vi "LibXML_GetNodeXMLText.vi"(8 "error in":errorcluster, 10 "xmlNodePtr":u32, 11 "xmlDocPtr":u32) -> (0 "error out":errorcluster, 3 "XMLString":string)   [LabVIEW 2019, in "Tools.lvlib"]
doc: "Gets the raw XML text of any node."
uses:
  Tools.lvlib
  dll/libxml2.dll
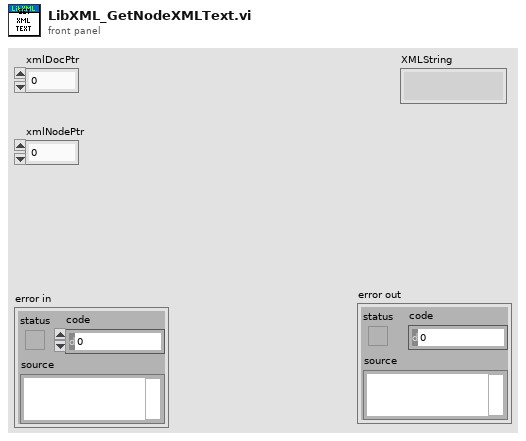
[diagram p1: front panel]
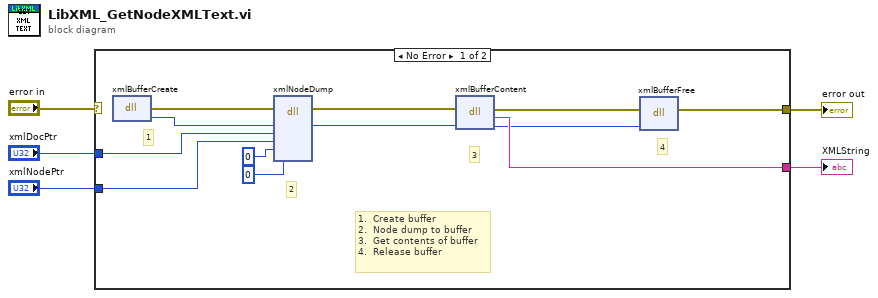
[diagram p0: block diagram]
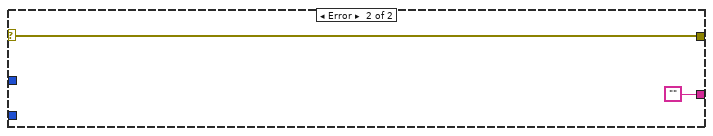
[diagram p2: hidden frame]
diagram:
  n1 = case shown="No Error" "error in" {
    selector: "error in" -> [_ w19]
    tunnel: "xmlDocPtr" -> [w15 _]
    tunnel: "xmlNodePtr" -> [w14 _]
    tunnel: [w11 ""] -> w3
    tunnel: [w6 w19] -> w2
    frame No Error {
      # "4"
      # "3"
      # "2"
      # "1"
      # "1.  Create buffer\n2.  Node dump to buffer\n3.  Get contents of buffer\n4.  Release buffer"
      n2 = dll-call lib="C:/Projects/_Prywatne/MyCIT/Framework/Tools/XML/LibXML/dll/libxml2.dll" fn="xmlBufferCreate"() -> (error out=w16:errorcluster, "xmlBufferPtr"=w17:u32)  [unwired: 3 in, 1 out]
      n3 = dll-call lib="C:/Projects/_Prywatne/MyCIT/Framework/Tools/XML/LibXML/dll/libxml2.dll" fn="xmlNodeDump"(error in=w16, "xmlBufferPtr"=w17, "xmlDocPtr"=w15, "xmlNodePtr"=w14, "level"=0, "format"=0) -> (error out=w12:errorcluster, "xmlBufferPtr"=w13:u32)  [unwired: 7 in, 1 out]
      n4 = dll-call lib="C:/Projects/_Prywatne/MyCIT/Framework/Tools/XML/LibXML/dll/libxml2.dll" fn="xmlBufferContent"(error in=w12, "xmlBufferPtr"=w13) -> (error out=w9:errorcluster, "XMLString"=w11:string, "xmlBufferPtr"=w10:u32)  [unwired: 2 in, 1 out]
      n5 = dll-call lib="C:/Projects/_Prywatne/MyCIT/Framework/Tools/XML/LibXML/dll/libxml2.dll" fn="xmlBufferFree"(error in=w9, "xmlBufferPtr"=w10) -> (error out=w6:errorcluster)  [unwired: 4 in, 1 out]
    }
    frame Error {
    }
  }
  "XMLString" <- w3
  "error out" <- w2
